vi "子VI-查看某框-不显示界面-只读穿透图模式.vi"(0 "框号":dbl format="%#_13g", 1 "框组":T3(array[cluster]), 2 "分层缺陷的面积阈值":i32, 3 "临界Z值":i32, 4 "弥散类缺陷灰度阈值":dbl caption="值", 5 "临界面积百分比值":dbl, 7 "预先配置的灰度阈值":dbl, 8 "穿透图原始路径":path, 9 "部位信息":string[](array[string])=["", "34.500000", "32.500000", "1121", "34", "54.955926", "分层类", "不合格", ""], 16 "产品规格":cluster{"产品长度（周长）（mm）":dbl, "产品宽度（母线长）（mm）":dbl}) -> (20 "全部检测结果":string[][](table))   [LabVIEW 2018]
uses:
  <vilib>/vision/NI_Vision_Development_Module.lvlib
panel:
  out "去掉的面积累计":dbl
  out "?":string[][](table)
  out "弥散类检测结果":string[][](table)
  out "中心Y":dbl
  out "中心X":dbl
  in  "格式字符串 4":string="%f"
  in  "分隔符（'\\'代码显示） 3":string="\t"
  in  "Tab Control":T1
  out "?":T2(plugin-control)
  out "Threshold Image":T2(plugin-control)
  out "Threshold Image":T2(plugin-control)
  in  "格式字符串 3":string="%f"
  in  "分隔符（'\\'代码显示） 2":string="\t"
  out "弥散和分层临界灰度值":i64
  out "弥散缺陷个数":i32
  out "分层缺陷个数":i32
  out "合格？ 弥散类":string="fencengThreshold"
  out "合格？分层类":string="fencengThreshold"
  out "弥散测量结果":i16[][](array[numeric])
  out "面积 (pixels)":i32
  in  "格式字符串 2":string="%f"
  in  "分隔符（'\\'代码显示）":string="\t"
  out "分层测量结果":i16[][](array[numeric])
  out "缺陷初步分类的临界值":sgl format="%#.3f"
  # "所选区域信息"
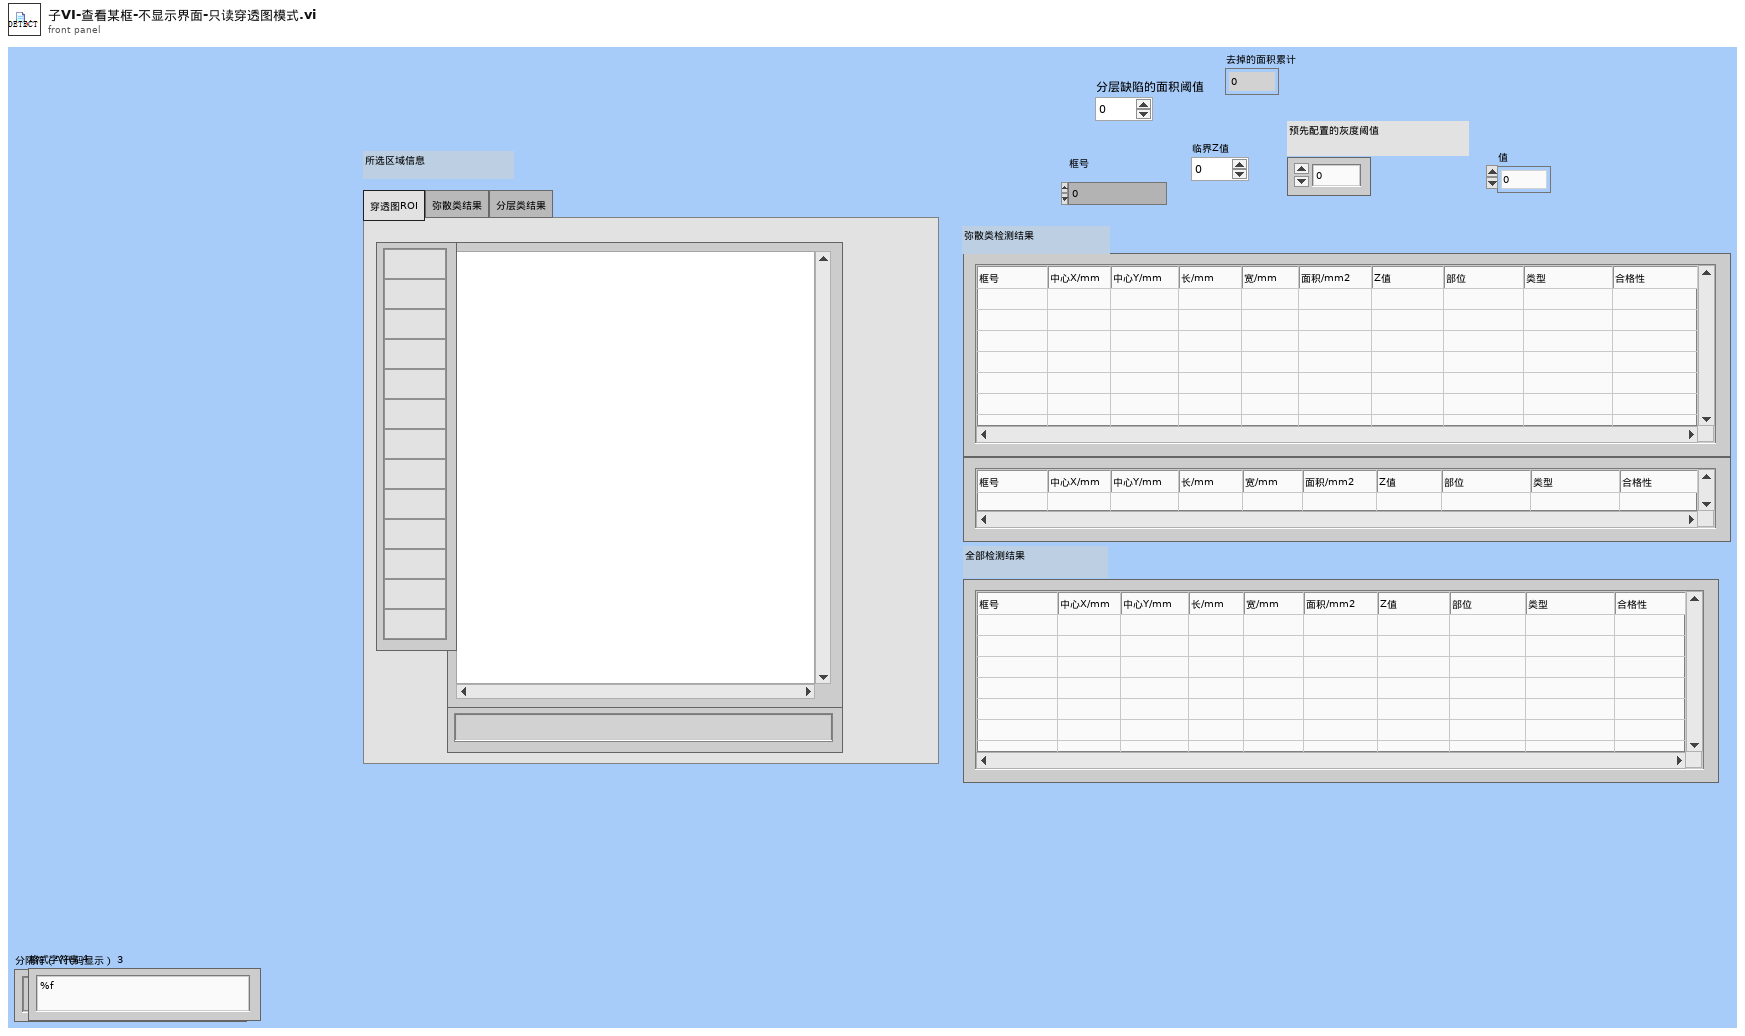
[diagram p1: front panel]
types:
  T1 = typedef "控件2.ctl" = enum32{"穿透图ROI", "弥散类结果", "分层类结果"}
  T2 = typedef "IMAQ Image.ctl" = refnum<image>
  T3 = cluster{"Global Rectangle":i32[], "Contours":cluster{"Contour Type":u32, "ROI Type":u32, "Points":i32[]}[]}[]
  T4 = typedef "Image Type" = u32
  T5 = typedef "Particle Parameters" = i32
  T6 = cluster{"Measurement Parameter":T5, "Range Lower Value":dbl, "Range Upper Value":dbl, "Range":bool, "Measurement Type":bool}[]
  T7 = cluster{"Global Rectangle":i32[], "Contours":cluster{"Contour Type":u32, "ROI Type":u32, "Points":i32[]}[]}
  T8 = cluster{"histogram":u32[], "Minimal Value":sgl, "Maximal Value":sgl, "Starting Value":sgl, "Interval Width":sgl, "Mean Value":sgl, "Standard  Variation":sgl, "Area (pixels)":i32}
  T9 = cluster{"Area":dbl, "Number of Holes":dbl, "Bounding Rect":cluster{"Left":dbl, "Top":dbl, "Right":dbl, "Bottom":dbl}, "Center of Mass":cluster{"X":dbl, "Y":dbl}, "Orientation":dbl, "Dimensions":cluster{"Width":dbl, "Height":dbl}}[]
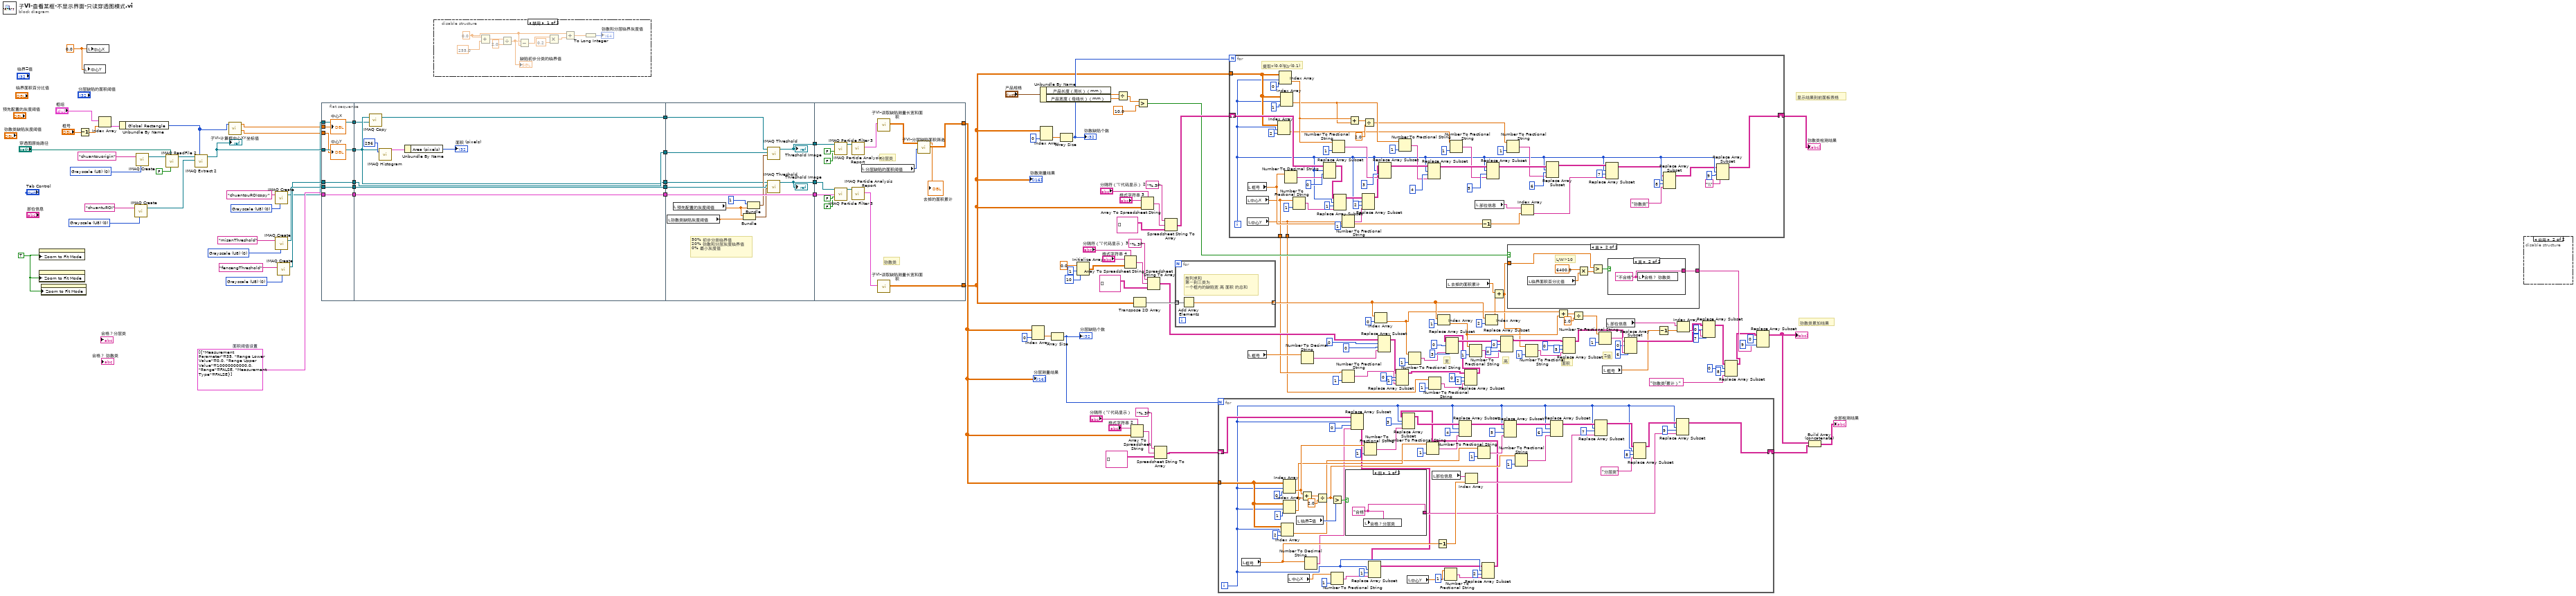
[diagram p0: block diagram]
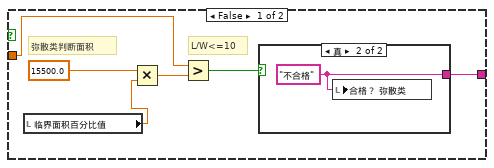
[diagram p3: hidden frame]
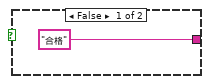
[diagram p4: hidden frame]
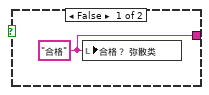
[diagram p5: hidden frame]
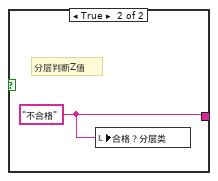
[diagram p6: hidden frame]
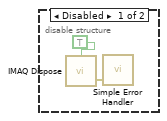
[diagram p7: hidden frame]
diagram:
  w6 = 0.0 ("中心X")
  w85 = T4 0 items=["Grayscale (U8)", "Grayscale (I16)", "Grayscale (SGL)", "Complex (CSG)", "RGB (U32)", "HSL (U32)", "RGB (U64)", "Grayscale (U16)"] ("Image Type")
  w90 = TRUE ("Zoom to Fit Mode")
  w124 = T4 0 items=["Grayscale (U8)", "Grayscale (I16)", "Grayscale (SGL)", "Complex (CSG)", "RGB (U32)", "HSL (U32)", "RGB (U64)", "Grayscale (U16)"] ("Image Type")
  w125 = T4 0 items=["Grayscale (U8)", "Grayscale (I16)", "Grayscale (SGL)", "Complex (CSG)", "RGB (U32)", "HSL (U32)", "RGB (U64)", "Grayscale (U16)"] ("Image Type")
  w128 = T4 0 items=["Grayscale (U8)", "Grayscale (I16)", "Grayscale (SGL)", "Complex (CSG)", "RGB (U32)", "HSL (U32)", "RGB (U64)", "Grayscale (U16)"] ("Image Type")
  w110 = T6 [{"Measurement Parameter"=35, "Range Lower Value"=0.0, "Range Upper Value"=10000000000.0, "Range"=FALSE, "Measurement Type"=FALSE}]  # 面积阈值设置
  w141 = T4 0 items=["Grayscale (U8)", "Grayscale (I16)", "Grayscale (SGL)", "Complex (CSG)", "RGB (U32)", "HSL (U32)", "RGB (U64)", "Grayscale (U16)"] ("Image Type")
  # "Z值"
  # "面积"
  # "高"
  # "宽"
  # "弥散类累加结果"
  # "显示结果到前面板表格"
  n1 = property class="ImageControl"("Zoom to Fit Mode"=w90) -> ()  [unwired: 2 in, 2 out]
  n2 = property class="ImageControl"("Zoom to Fit Mode"=w90) -> ()  [unwired: 2 in, 2 out]
  n3 = property class="ImageControl"("Zoom to Fit Mode"=w90) -> ()  [unwired: 2 in, 2 out]
  n4 = Decrement(x="框号") -> (x-1=w143:dbl)
  n5 = local write "中心Y"(w6) -> ()
  n6 = local write "中心X"(w6) -> ()
  n7 = Index Array(array="框组", index=w143) -> (element=w144:T7)
  n8 = Unbundle By Name(w144) -> ("Global Rectangle"=w33:i32[])
  n9 = call "IMAQ Create"("Image Name"="chuantuROI", "Image Type"=w128) -> ("New Image"=w127:T2)  [unwired: 3 in, 1 out]
  n10 = call "IMAQ Create"("Image Name"="chuantouorigin", "Image Type"=w141) -> ("New Image"=w130:T2)  [unwired: 3 in, 1 out]
  n11 = call "IMAQ ReadFile 2"("Use File Path Image Type"=FALSE, "File Path"="穿透图原始路径", "Image"=w130) -> ("Image Out"=w131:T2)  [unwired: 4 in, 4 out]
  n12 = call "IMAQ Extract 2"("Optional Rectangle"=w33, "Image Dst"=w127, "Image Src"=w131) -> ("Image Dst Out"=w93:T2)  [unwired: 7 in, 1 out]
  "?" <- w93
  n13 = call "子VI-计算框中心XY坐标值.vi"("Global Rectangle"=w33) -> ("中心Y"=w7:dbl, "中心X"=w8:dbl)  [unwired: 9 in]
  n14 = call "IMAQ Create"("Image Name"="chuantouROIcopy", "Image Type"=w85) -> ("New Image"=w88:T2)  [unwired: 3 in, 1 out]
  n15 = call "IMAQ Create"("Image Name"="misanThreshold", "Image Type"=w124) -> ("New Image"=w117:T2)  [unwired: 3 in, 1 out]
  n16 = call "IMAQ Create"("Image Name"="fencengThreshold", "Image Type"=w125) -> ("New Image"=w115:T2)  [unwired: 3 in, 1 out]
  n17 = flat-sequence {
    tunnel: w93 -> [w150]
    tunnel: w117 -> [w153]
    tunnel: [w153] -> w118
    tunnel: [w152] -> w116
    tunnel: w115 -> [w152]
    tunnel: [w151] -> w111
    tunnel: w110 -> [w151]
    tunnel: [w150] -> w91
    tunnel: w88 -> [w149]
    tunnel: [w149] -> w87
    tunnel: w8 -> [w148]
    tunnel: w7 -> [w147]
    tunnel: [w162] -> w119
    tunnel: [w161] -> w114
    tunnel: [w157] -> w109
    tunnel: w111 -> [w157]
    tunnel: w116 -> [w161]
    tunnel: w118 -> [w162]
    tunnel: [w156] -> w92
    tunnel: w91 -> [w156]
    tunnel: [w155] -> w89
    tunnel: w87 -> [w154]
    tunnel: w119 -> [w174]
    tunnel: w114 -> [w173]
    tunnel: [w167] -> w113
    tunnel: [w168] -> w112
    tunnel: w109 -> [w172]
    tunnel: [w172] -> w108
    tunnel: w92 -> [w169]
    tunnel: w89 -> [w166]
    tunnel: [w181] -> w75
    tunnel: [w176] -> w101
    tunnel: w113 -> [w184]
    tunnel: w112 -> [w185]
    tunnel: w108 -> [w188]
    frame #0 {
      "中心X" <- w148
      "中心Y" <- w147
    }
    frame #1 {
      n18 = call "IMAQ Copy"("Image Dst"=w154, "Image Src"=w156) -> ("Image Dst Out"=w155:T2)  [unwired: 4 in, 1 out]
      n19 = call "IMAQ Histogram"("Number of Classes"=256, "Image"=w156) -> ("Histogram Report"=w159:T8)  [unwired: 8 in, 1 out]
      n20 = Unbundle By Name(w159) -> ("Area (pixels)"=→"面积 (pixels)":i32)
    }
    frame #2 {
      # "50% 初步分类临界值\n20% 弥散和分层灰度临界值\n0% 最小灰度值"
      n21 = local read "弥散类缺陷灰度阈值"() -> (w163:dbl)
      n22 = local read "预先配置的灰度阈值"() -> (w164:dbl)
      n23 = Bundle("预先配置的灰度阈值"=w164, "弥散类缺陷灰度阈值"=w163) -> (w171:cluster{"预先配置的灰度阈值":dbl, "弥散类缺陷灰度阈值":dbl})  [unwired: 1 in]
      n24 = Bundle(1, "预先配置的灰度阈值"=w164) -> (w170:cluster{i32, "预先配置的灰度阈值":dbl})  [unwired: 1 in]
      n25 = call "IMAQ Threshold"("Range"=w170, "Image Dst"=w173, "Image Src"=w166) -> ("Image Dst Out"=w167:T2)  [unwired: 3 in, 5 out]
      "Threshold Image" <- w167
      n26 = call "IMAQ Threshold"("Range"=w171, "Image Dst"=w174, "Image Src"=w169) -> ("Image Dst Out"=w168:T2)  [unwired: 3 in, 5 out]
      "Threshold Image" <- w168
    }
    frame #3 {
      # "分层类"
      # "弥散类"
      n27 = call "IMAQ Particle Filter 3"("Image Src"=w184, "Keep/Remove Particles (F)"=FALSE, "Reject Border? (F)"=FALSE) -> ("Image Dst Out"=w183:T2)  [unwired: 10 in, 2 out]
      n28 = call "IMAQ Particle Filter 3"("Image Src"=w185, "Selection Values"=w188, "Keep/Remove Particles (F)"=FALSE, "Reject Border? (F)"=FALSE) -> ("Image Dst Out"=w179:T2)  [unwired: 9 in, 2 out]
      n29 = call "IMAQ Particle Analysis Report"("Image"=w183) -> ("Particle Reports (Pixels)"=w182:T9)  [unwired: 5 in, 5 out]
      n30 = call "IMAQ Particle Analysis Report"("Image"=w179) -> ("Particle Reports (Pixels)"=w180:T9)  [unwired: 5 in, 5 out]
      n31 = local read "分层缺陷的面积阈值"() -> (w177:i32)
      n32 = call "子VI-读取缺陷测量长宽和面积.vi"("Particle Reports (Pixels)"=w182) -> ("测量结果"=w178:dbl[][])  [unwired: 10 in]
      n33 = call "子VI-读取缺陷测量长宽和面积.vi"("Particle Reports (Pixels)"=w180) -> ("测量结果"=w181:dbl[][])  [unwired: 10 in]
      n34 = call "子VI-分层缺陷面积筛选.vi"("计入分层缺陷的面积阈值"=w177, "分层测量结果"=w178) -> ("初始化的数组"=w176:dbl[][], "去掉的面积累计"=→"去掉的面积累计":dbl)  [unwired: 8 in]
    }
  }
  n35 = disable-structure shown="禁用" {
    frame Disabled {
      w194 = sgl 0.0 ("x")
      n36 = Add(x=w194, y=sgl 255.0) -> (x+y=w196:sgl)
      n37 = Divide(x=w196, y=sgl 2.0) -> (x/y=w197:sgl)
      "缺陷初步分类的临界值" <- w197
      n38 = Subtract(x=w197, y=w194) -> (x-y=w198:sgl)
      n39 = Multiply(x=w198, y=0.2) -> (x*y=w199:dbl)
      n40 = Add(x=w194, y=w199) -> (x+y=w200:dbl)
      n41 = To Long Integer(number=w200) -> (32bit integer=→"弥散和分层临界灰度值":i32)
    }
    frame Enabled {
    }
  }
  n42 = Index Array(array=w101, index (col)=0 ("禁用的索引 (列)")) -> (element=w123:dbl[])  [unwired: 1 in]
  n43 = Unbundle By Name("产品规格") -> ("产品长度（周长）（mm）"=w135:dbl, "产品宽度（母线长）（mm）"=w134:dbl)
  n44 = Index Array(array=w75, index (col)=0 ("禁用的索引 (列)")) -> (element=w121:dbl[])  [unwired: 1 in]
  n45 = Array Size(array=w123) -> (size(s)=w107:i32)
  "分层缺陷个数" <- w107
  n46 = Array Size(array=w121) -> (size(s)=w133:i32)
  "弥散缺陷个数" <- w133
  n47 = Initialize Array(0.0 ("元素"), 1 ("维数大小"), 10 ("维数大小")) -> (w76:dbl[][])
  n48 = Divide(x=w135, y=w134) -> (x/y=w138:dbl)
  n49 = Array To Spreadsheet String(delimiter (Tab)="分隔符（'\\'代码显示） 3", array=w76, 3:"格式字符串 4") -> (spreadsheet string=w79:string)
  n50 = Array To Spreadsheet String(delimiter (Tab)="分隔符（'\\'代码显示）", array=w101, 3:"格式字符串 2") -> (spreadsheet string=w104:string)
  n51 = Transpose 2D Array(2D array=w75) -> (transposed array=w74:dbl[][])
  n52 = Greater?(x=w138, y=10.0) -> (0:w38:bool)
  n53 = Array To Spreadsheet String(delimiter (Tab)="分隔符（'\\'代码显示） 2", array=w75, 3:"格式字符串 3") -> (spreadsheet string=w97:string)
  n54 = Spreadsheet String To Array(format string="%.3f", spreadsheet string=w79, array type (2D Dbl)=string[][] [] ("Array")) -> (array=w37:string[][])  [unwired: 1 in]
  n55 = Spreadsheet String To Array(format string="%.3f", spreadsheet string=w104, array type (2D Dbl)=string[][] [] ("Array")) -> (array=w100:string[][])  [unwired: 1 in]
  n56 = Spreadsheet String To Array(format string="%.3f", spreadsheet string=w97, array type (2D Dbl)=string[][] [] ("Array")) -> (array=w94:string[][])  [unwired: 1 in]
  n57 = for {
    tunnel: w74 -> [w202] mode=indexing
    tunnel: [w201] -> w41 mode=indexing
    # "按列求和 \n第一到三类为\n一个框内的缺陷宽 高 面积 的总和"
    n58 = Add Array Elements(numeric array=w202) -> (sum=w201:dbl)
  }
  n59 = for {
    N: w107 -> [_]
    tunnel: w101 -> [w225]
    shift-right: [w233] -> w35
    shift-left: w100 -> [w241]
    i -> [w210]
    n60 = local read "框号"() -> (w248:dbl)
    n61 = Index Array(array=w225, index (row)=w210, index (col)=2 ("索引 (列)")) -> (element=w224:dbl)
    n62 = Index Array(array=w225, index (row)=w210, index (col)=0 ("禁用的索引 (列)")) -> (element=w232:dbl)
    n63 = Index Array(array=w225, index (row)=w210, index (col)=1 ("禁用的索引 (列)")) -> (element=w231:dbl)
    n64 = local read "中心X"() -> (w217:dbl)
    n65 = local read "临界Z值"() -> (w255:i32)
    n66 = Add(x=w232, y=w231) -> (x+y=w256:dbl)
    n67 = Number To Decimal String(number=w248) -> (decimal integer string=w223:string)  [unwired: 1 in]
    n68 = Divide(x=w256, y=2.0) -> (x/y=w229:dbl)
    n69 = Number To Fractional String(number=w217, precision (6)=i16 1 ("精度(6)")) -> (F-format string=w216:string)  [unwired: 2 in]
    n70 = Greater?(x=w229, y=w255) -> (0:w257:bool)
    n71 = case shown="假" w257 {
      tunnel: [w258 w259] -> w227
      frame False {
        w258 = "合格" ("合格？")
        n72 = local write "合格？分层类"(w258) -> ()
      }
      frame True {
        w259 = "不合格" ("合格？")
        # "分层判断Z值"
        n73 = local write "合格？分层类"(w259) -> ()
      }
    }
    n74 = Replace Array Subset(array=w241, new element=w223, index (row)=w210, index (col)=0 ("索引 (列)")) -> (w208:string[][])
    n75 = Number To Fractional String(number=w232, precision (6)=i16 1 ("精度(6)")) -> (F-format string=w240:string)  [unwired: 2 in]
    n76 = Replace Array Subset(array=w208, new element=w216, index (row)=w210, index (col)=1 ("索引 (列)")) -> (w209:string[][])
    n77 = local read "中心Y"() -> (w214:dbl)
    n78 = Number To Fractional String(number=w231, precision (6)=i16 1 ("精度(6)")) -> (F-format string=w239:string)  [unwired: 2 in]
    n79 = local read "部位信息"() -> (w251:string[])
    n80 = Decrement(x=w248) -> (x-1=w250:dbl)
    n81 = Number To Fractional String(number=w214, precision (6)=i16 1 ("精度(6)")) -> (F-format string=w212:string)  [unwired: 2 in]
    n82 = Index Array(array=w251, index=w250) -> (element=w228:string)
    n83 = Number To Fractional String(number=w224, precision (6)=i16 1 ("精度(6)")) -> (F-format string=w236:string)  [unwired: 2 in]
    n84 = Replace Array Subset(array=w209, new element=w212, index (row)=w210, index (col)=2 ("索引 (列)")) -> (w207:string[][])
    n85 = Replace Array Subset(array=w207, new element=w240, index (row)=w210, index (col)=3 ("索引 (列)")) -> (w238:string[][])
    n86 = Replace Array Subset(array=w238, new element=w239, index (row)=w210, index (col)=4 ("索引 (列)")) -> (w237:string[][])
    n87 = Replace Array Subset(array=w237, new element=w236, index (row)=w210, index (col)=5 ("索引 (列)")) -> (w235:string[][])
    n88 = Number To Fractional String(number=w229, precision (6)=i16 1 ("精度(6)")) -> (F-format string=w230:string)  [unwired: 2 in]
    n89 = Replace Array Subset(array=w235, new element=w230, index (row)=w210, index (col)=6 ("索引 (列)")) -> (w234:string[][])
    n90 = Replace Array Subset(array=w234, new element=w228, index (row)=w210, index (col)=7 ("索引 (列)")) -> (w222:string[][])
    n91 = Replace Array Subset(array=w222, new element="分层类" ("新元素/子数组"), index (row)=w210, index (col)=8 ("禁用的索引 (列)")) -> (w219:string[][])
    n92 = Replace Array Subset(array=w219, new element=w227, index (row)=w210, index (col)=9 ("索引 (列)")) -> (w233:string[][])
  }
  n93 = for {
    N: w133 -> [_]
    tunnel: w75 -> [w284]
    shift-right: [w298] -> w32
    shift-left: w94 -> [w303]
    tunnel: [w261] -> w5
    tunnel: [w260] -> w4
    i -> [w269]
    # "提取x(0,0)和y(0,1)"
    n94 = local read "中心X"() -> (w261:dbl)
    n95 = local read "中心Y"() -> (w260:dbl)
    n96 = local read "框号"() -> (w286:dbl)
    n97 = Index Array(array=w284, index (row)=w269, index (col)=2 ("禁用的索引 (列)")) -> (element=w282:dbl)
    n98 = Index Array(array=w284, index (row)=w269, index (col)=0 ("禁用的索引 (列)")) -> (element=w292:dbl)
    n99 = Index Array(array=w284, index (row)=w269, index (col)=1 ("禁用的索引 (列)")) -> (element=w291:dbl)
    n100 = Number To Decimal String(number=w286) -> (decimal integer string=w280:string)  [unwired: 1 in]
    n101 = Number To Fractional String(number=w261, precision (6)=i16 1 ("精度(6)")) -> (F-format string=w277:string)  [unwired: 2 in]
    n102 = Replace Array Subset(array=w303, new element=w280, index (row)=w269, index (col)=0 ("索引 (列)")) -> (w274:string[][])
    n103 = Number To Fractional String(number=w292, precision (6)=i16 1 ("精度(6)")) -> (F-format string=w297:string)  [unwired: 2 in]
    n104 = Replace Array Subset(array=w274, new element=w277, index (row)=w269, index (col)=1 ("索引 (列)")) -> (w273:string[][])
    n105 = Number To Fractional String(number=w260, precision (6)=i16 1 ("精度(6)")) -> (F-format string=w271:string)  [unwired: 2 in]
    n106 = Add(x=w292, y=w291) -> (x+y=w294:dbl)
    n107 = Replace Array Subset(array=w273, new element=w271, index (row)=w269, index (col)=2 ("索引 (列)")) -> (w272:string[][])
    n108 = Divide(x=w294, y=2.0) -> (x/y=w290:dbl)
    n109 = Replace Array Subset(array=w272, new element=w297, index (row)=w269, index (col)=3 ("索引 (列)")) -> (w302:string[][])
    n110 = Number To Fractional String(number=w291, precision (6)=i16 1 ("精度(6)")) -> (F-format string=w296:string)  [unwired: 2 in]
    n111 = Replace Array Subset(array=w302, new element=w296, index (row)=w269, index (col)=4 ("索引 (列)")) -> (w301:string[][])
    n112 = Number To Fractional String(number=w282, precision (6)=i16 1 ("精度(6)")) -> (F-format string=w295:string)  [unwired: 2 in]
    n113 = local read "部位信息"() -> (w288:string[])
    n114 = Decrement(x=w286) -> (x-1=w287:dbl)
    n115 = Replace Array Subset(array=w301, new element=w295, index (row)=w269, index (col)=5 ("索引 (列)")) -> (w300:string[][])
    n116 = Number To Fractional String(number=w290, precision (6)=i16 1 ("精度(6)")) -> (F-format string=w289:string)  [unwired: 2 in]
    n117 = Index Array(array=w288, index=w287) -> (element=w285:string)
    n118 = Replace Array Subset(array=w300, new element=w289, index (row)=w269, index (col)=6 ("索引 (列)")) -> (w299:string[][])
    n119 = Replace Array Subset(array=w299, new element=w285, index (row)=w269, index (col)=7 ("索引 (列)")) -> (w267:string[][])
    n120 = Replace Array Subset(array=w267, new element="弥散类" ("新元素/子数组"), index (row)=w269, index (col)=8 ("索引 (列)")) -> (w266:string[][])
    n121 = Replace Array Subset(array=w266, new element="\\" ("新元素/子数组"), index (row)=w269, index (col)=9 ("索引 (列)")) -> (w298:string[][])
  }
  "弥散类检测结果" <- w32
  n122 = local read "框号"() -> (w36:dbl)
  n123 = Number To Decimal String(number=w36) -> (decimal integer string=w25:string)  [unwired: 1 in]
  n124 = Number To Fractional String(number=w5, precision (6)=i16 1 ("精度(6)")) -> (F-format string=w18:string)  [unwired: 2 in]
  n125 = Index Array(array=w41, index=0 ("索引")) -> (element=w40:dbl)
  n126 = Replace Array Subset(array=w37, new element=w25, index (row)=0 ("禁用的索引 (行)"), index (col)=0 ("索引 (列)")) -> (w15:string[][])
  n127 = Replace Array Subset(array=w15, new element=w18, index (row)=0 ("索引 (行)"), index (col)=1 ("索引 (列)")) -> (w14:string[][])
  n128 = Number To Fractional String(number=w40, precision (6)=i16 1 ("精度(6)")) -> (F-format string=w68:string)  [unwired: 2 in]
  n129 = Number To Fractional String(number=w4, precision (6)=i16 1 ("精度(6)")) -> (F-format string=w16:string)  [unwired: 2 in]
  n130 = Index Array(array=w41, index=1 ("索引")) -> (element=w39:dbl)
  n131 = local read "去掉的面积累计"() -> (w2:dbl)
  n132 = Replace Array Subset(array=w14, new element=w16, index (row)=0 ("索引 (行)"), index (col)=2 ("索引 (列)")) -> (w13:string[][])
  n133 = Replace Array Subset(array=w13, new element=w68, index (row)=0 ("索引 (行)"), index (col)=3 ("索引 (列)")) -> (w66:string[][])
  n134 = Number To Fractional String(number=w39, precision (6)=i16 1 ("精度(6)")) -> (F-format string=w59:string)  [unwired: 2 in]
  n135 = Index Array(array=w41, index=2 ("索引")) -> (element=w3:dbl)
  n136 = Add(x=w2, y=w3) -> (x+y=w1:dbl)
  n137 = Replace Array Subset(array=w66, new element=w59, index (row)=0 ("索引 (行)"), index (col)=4 ("禁用的索引 (列)")) -> (w61:string[][])
  n138 = case shown="真" w38 {
    tunnel: [w317 w325] -> w42
    tunnel: w1 -> [w313 w321]
    frame False {
      # "弥散类判断面积"
      # "L/W<=10"
      n139 = local read "临界面积百分比值"() -> (w314:dbl)
      n140 = Multiply(x=15500.0, y=w314) -> (x*y=w315:dbl)
      n141 = Greater?(x=w313, y=w315) -> (0:w318:bool)
      n142 = case shown="真" w318 {
        tunnel: ["合格" ("合格？") w320] -> w317
        frame False {
        }
        frame True {
          w320 = "不合格" ("合格？")
          n143 = local write "合格？ 弥散类"(w320) -> ()
        }
      }
    }
    frame True {
      # "L/W>10"
      n144 = local read "临界面积百分比值"() -> (w322:dbl)
      n145 = Multiply(x=6400.0, y=w322) -> (x*y=w324:dbl)
      n146 = Greater?(x=w321, y=w324) -> (0:w326:bool)
      n147 = case shown="真" w326 {
        tunnel: [w327 w328] -> w325
        frame False {
          w327 = "合格" ("合格？")
          n148 = local write "合格？ 弥散类"(w327) -> ()
        }
        frame True {
          w328 = "不合格" ("合格？")
          n149 = local write "合格？ 弥散类"(w328) -> ()
        }
      }
    }
  }
  n150 = Number To Fractional String(number=w1, precision (6)=i16 1 ("精度(6)")) -> (F-format string=w58:string)  [unwired: 2 in]
  n151 = Add(x=w40, y=w39) -> (x+y=w57:dbl)
  n152 = Replace Array Subset(array=w61, new element=w58, index (row)=0 ("索引 (行)"), index (col)=5 ("索引 (列)")) -> (w51:string[][])
  n153 = Divide(x=w57, y=2.0) -> (x/y=w55:dbl)
  n154 = Number To Fractional String(number=w55, precision (6)=i16 1 ("精度(6)")) -> (F-format string=w54:string)  [unwired: 2 in]
  n155 = local read "框号"() -> (w34:dbl)
  n156 = local read "部位信息"() -> (w49:string[])
  n157 = Replace Array Subset(array=w51, new element=w54, index (row)=0 ("索引 (行)"), index (col)=6 ("索引 (列)")) -> (w45:string[][])
  n158 = Decrement(x=w34) -> (x-1=w50:dbl)
  n159 = Index Array(array=w49, index=w50) -> (element=w48:string)
  n160 = Replace Array Subset(array=w45, new element=w48, index (row)=0 ("索引 (行)"), index (col)=7 ("索引 (列)")) -> (w27:string[][])
  n161 = Replace Array Subset(array=w27, new element="弥散类(累计）" ("新元素/子数组"), index (row)=0 ("索引 (行)"), index (col)=8 ("索引 (列)")) -> (w26:string[][])
  n162 = Replace Array Subset(array=w26, new element=w42, index (row)=0 ("索引 (行)"), index (col)=9 ("索引 (列)")) -> (w30:string[][])
  "?" <- w30
  n163 = Build Array (concatenate)(w30, w35) -> (→"全部检测结果":string[][])
  n164 = disable-structure shown="启用" {
    frame Disabled {
      n165 = call "IMAQ Dispose"("All Images? (No)"=TRUE) -> ("error out"=w330:errorcluster)  [unwired: 5 in]
      n166 = call <vilib>:"Simple Error Handler.vi"("error in (no error)"=w330) -> ()  [unwired: 4 in, 5 out]
    }
    frame Enabled {
    }
  }
  "分层测量结果" <- w101
  "弥散测量结果" <- w75
